vi "ep_Cross Judge.vi"(7 "over threshold?":bool, 9 "over index?":bool, 10 "y2":dbl, 11 "y1":dbl) -> (2 "cross":bool)   [LabVIEW 2012, in "NI_EP_Resample_Host.lvlib"]
uses:
  <vilib>/addons/Electrical Power/PQ/Resampling/NI_EP_Resample_Host.lvlib
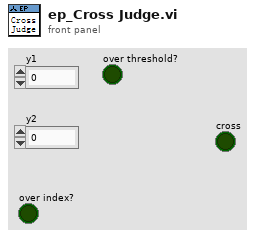
[diagram p1: front panel]
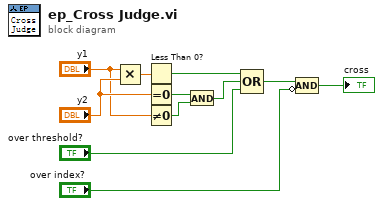
[diagram p0: block diagram]
diagram:
  n1 = Multiply(x="y1", y="y2") -> (x*y=w11:dbl)
  n2 = Less Than 0?(x=w11) -> (x < 0?=w5:bool)
  n3 = Equal To 0?(x="y2") -> (x = 0?=w7:bool)
  n4 = Not Equal To 0?(x="y1") -> (x != 0?=w8:bool)
  n5 = And(x=w7, y=w8) -> (x .and. y?=w6:bool)
  n6 = Compound Arithmetic op=OR(w5, w6, "over threshold?") -> (w4:bool)
  n7 = Compound Arithmetic op=AND(w4, invert "over index?") -> (→"cross":bool)
